vi "Set Error Message.vi"(4 "enable":bool=TRUE, 5 "error in":errorcluster, 7 "code":i32=-1, 8 "message":string="User error message.") -> (0 "error out":errorcluster {"code" format="%.0x"})   [LabVIEW 2010]
doc: "If enabled (default), set the error status, code, and message values."
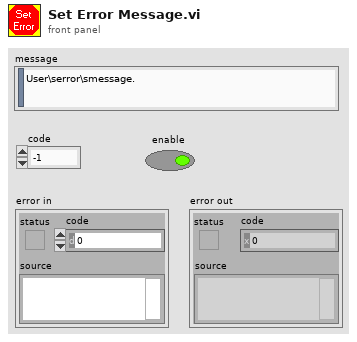
[diagram p1: front panel]
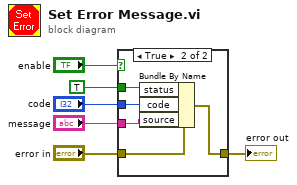
[diagram p0: block diagram]
diagram:
  n1 = case shown="True" "enable" {
    tunnel: "code" -> [_ w12]
    tunnel: TRUE ("status") -> [_ w11]
    tunnel: "message" -> [_ w10]
    tunnel: "error in" -> [w7 w9]
    tunnel: [w7 w8] -> w2
    frame False {
    }
    frame True {
      n2 = Bundle By Name(cluster=w9, "status"=w11, "code"=w12, "source"=w10) -> (w8:errorcluster)
    }
  }
  "error out" <- w2
